vi "Write DB.vi"(8 "error in (no error)":errorcluster, 10 "Database.lvlib:Database.lvclass":refnum<class "Database.lvclass">, 11 "Panel Form Controller in":refnum<class "Panel Form Controller.lvclass">) -> (0 "error out":errorcluster, 3 "Panel Form Controller out":refnum<class "Panel Form Controller.lvclass">)   [LabVIEW 2020, in "Panel Form Controller.lvlib" / "Panel Form Controller.lvclass"]
uses:
  Panel Form Controller.lvclass
  Database OOP/Database/Database Class/Database.lvclass
  Panel Form Controller.lvclass/Panel Form Controller.ctl
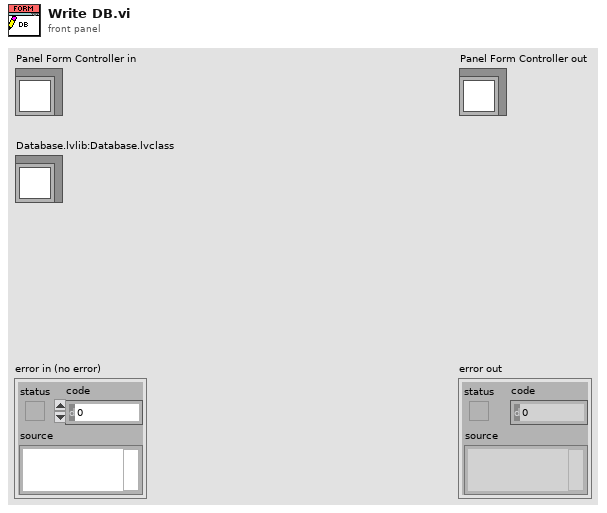
[diagram p1: front panel]
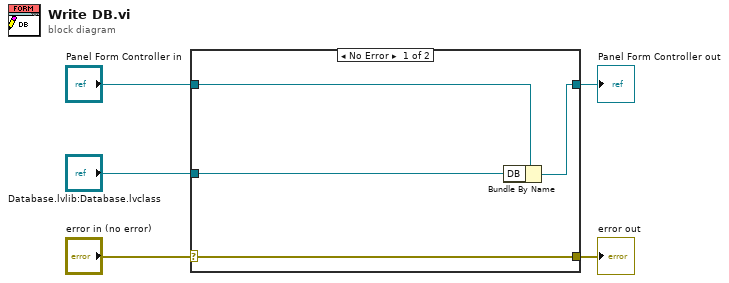
[diagram p0: block diagram]
diagram:
  n1 = case shown="No Error" "error in (no error)" {
    selector: "error in (no error)" -> [w9 w10]
    tunnel: [w9 w10] -> w4
    tunnel: [w7 w11] -> w2
    tunnel: "Panel Form Controller in" -> [w8 w11]
    tunnel: "Database.lvlib:Database.lvclass" -> [w6 _]
    frame No Error {
      n2 = Bundle By Name(cluster=w8, "DB"=w6) -> (w7:refnum<class "Panel Form Controller.lvclass">)
    }
    frame Error {
    }
  }
  "error out" <- w4
  "Panel Form Controller out" <- w2
